vi "WVDIAL_1_AMCS_3.0.vi"() -> ()   [LabVIEW 2012]
uses:
  <vilib>/Analysis/baseanly.llb/Mean (DBL).vi
  NCAR_DIAL_Labview/AMCS_Data.vi
  AmcsUsb.dll
  <vilib>/Analysis/NI_AALBase.lvlib
panel:
  in  "scalar wait time (remove at some point)":i32=550
  in  "channel":i32=1
  in  "CH mult":dbl=1.0
  out "size(s)":i32=2241
  in  "Channels":u32=4
  in  "Data Reads":i32=52
  out "Loop Count":i32=52
  in  "TC Start":i32=2 min=1 max=1894
  in  "TC Length":i32=15 min=2 max=280
  out "TC background sub over length":cluster{dbl, dbl, dbl, dbl}(graph)={5109.382978723404, 7254.3829787234035, 34.71276595744666, -41.031914893617085}
  out "return type":i32
  out "Raw Uncorrected Return":u16[][](graph)=[[23170, 208, 128, 150, 143, 140, 160, 194, 234, 298, 421, 538, 627, 660, 684, 718, 683, 714, 813, 891, 935, 839, 807, 607, 402, 336, 228, 191, 162, 179, 228, 223, 180, 171, 156, 120, 118, 147, 143, 128, 135, 133, 141, 169, 169, 196, 157, 140, 161, 341, 3035, 18784, 23099, 23731, 21071, 6231, 426, 67, 48, 46, 51, 41, 49, 50, 54, 60, 46, 47, 40, 38, 53, 40, 37, 41, 51, 45, 57, 38, 34, 35, 35, 47, 51, 51, 57, 49, 51, 52, 33, 45, 62, 49, 34, 47, 42, 44, 35, 55, 54, 36, 40, 34, 41, 56, 52, 37, 44, 51, 52, 37, 54, 57, 45, 32, 35, 55, 44, 57, 40, 38, 37, 51, 48, 35, 55, 35, 43, 47, 48, 34, 44, 54, 44, 55, 51, 38, 46, 50, 51, 37, 44, 45, 40, 52, 42, 40, 55, 45, 40, 44, 44, 46, 38, 45, 53, 40, 52, 46, 52, 46, 42, 39, 43, 41, 34, 32, 30, 45, 46, 47, 44, 46, 37, 46, 36, 45, 49, 50, 42, 38, 45, 42, 46, 49, 51, 50, 40, 51, 36, 36, 46, 45, 37, 53, 48, 55, 51, 48, 41, 36, 47, 39, 36, 36, 36, 46, 44, 46, 43, 41, 39, 51, 51, 43, 50, 42, 44, 41, 44, 53, 54, 37, 52, 46, 46, 37, 40, 44, 42, 48, 39, 61, 40, 43, 41, 47, 42, 42, 38, 47, 34, 45, 40, 34, 44, 39, 48, 37, 53, 44, 54, 54, 48, 61, 42, 55, 39, 34, 34, 38, 38, 47, 54, 49, 44, 46, 39, 53, 49, 51, 32, 46, 39, 54, 53, 49, 34, 56, 47, 41, 47, 40, 40, 42, 34, 43, 55, 49, 47, 41, 51, 56, 63, 54, 47, 47, 44, 56, 38, 63, 42, 56, 62, 47, 37, 50, 59, 50, 42, 51, 53, 47, 43, 64, 40, 28, 41, 46, 27, 33, 56, 46, 57, 46, 58, 39, 55, 49, 49, 37, 58, 43, 38, 49, 47, 47, 33, 45, 45, 53, 42, 50, 49, 39, 43, 40, 44, 43, 49, 48, 44, 37, 42, 46, 52, 49, 45, 41, 44, 45, 36, 54, 50, 37, 34, 41, 40, 44, 37, 41, 45, 43, 56, 42, 40, 40, 34, 57, 39, 37, 42, 33, 46, 35, 40, 39, 40, 61, 38, 67, 32, 46, 61, 46, 46, 35, 42, 40, 50, 54, 47, 45, 41, 49, 47, 41, 49, 34, 46, 39, 50, 54, 45, 43, 54, 45, 50, 55, 46, 40, 37, 41, 34, 41, 46, 50, 44, 37, 55, 40, 41, 38, 37, 45, 45, 37, 37, 58, 51, 50, 39, 43, 50, 57, 49, 54, 52, 46, 43, 51, 47, 52, 45, 41, 52, 60, 51, 57, 42, 31, 46, 39, 33, 48, 42, 52, 49, 44, 51, 44, 49, 44, 39, 56, 42, 48, 41, 40, 45, 45, 40, 52, 40, 39, 38, 45, 41, 29, 44, 40, 41, 46, 50, 49, 23, 49, 52, 50, 50, 51, 50, 49, 46, 50, 39, 38, 49, 39, 50, 41, 40, 46, 36, 46, 51, 42, 37, 56, 37, 33, 43, 47, 56, 42, 48, 40, 45, 45, 49, 39, 51, 41, 43, 56, 31, 52, 35, 39, 52, 40, 44, 53, 30, 42, 48, 57, 43, 45, 39, 45, 47, 41, 52, 44, 50, 43, 52, 47, 46, 47], [23369, 189, 136, 142, 167, 134, 179, 206, 287, 391, 570, 714, 901, 981, 1009, 1038, 1068, 1177, 1297, 1480, 1537, 1540, 1386, 1167, 790, 593, 416, 343, 403, 448, 437, 400, 357, 324, 341, 292, 279, 332, 328, 343, 302, 341, 351, 440, 450, 458, 412, 358, 375, 976, 9005, 41499, 46820, 47461, 45458, 18218, 1558, 164, 60, 56, 54, 51, 52, 44, 56, 44, 48, 43, 44, 39, 37, 55, 38, 44, 44, 36, 58, 48, 44, 41, 49, 40, 50, 43, 41, 40, 46, 40, 41, 48, 55, 41, 48, 32, 47, 62, 38, 44, 40, 39, 56, 35, 37, 44, 39, 35, 33, 50, 45, 45, 43, 46, 46, 48, 41, 44, 37, 44, 49, 35, 40, 48, 55, 53, 57, 45, 43, 53, 51, 42, 46, 42, 52, 49, 46, 57, 38, 43, 52, 40, 33, 41, 46, 51, 40, 43, 42, 53, 41, 42, 42, 38, 52, 46, 43, 34, 40, 47, 43, 44, 50, 48, 45, 34, 33, 35, 46, 36, 50, 30, 51, 55, 54, 43, 41, 47, 47, 45, 57, 38, 47, 46, 58, 53, 48, 53, 45, 42, 50, 37, 52, 40, 41, 53, 57, 47, 46, 49, 46, 37, 50, 41, 38, 47, 49, 43, 58, 49, 44, 40, 41, 47, 50, 35, 47, 50, 42, 51, 29, 48, 46, 57, 34, 43, 51, 45, 47, 52, 33, 45, 46, 32, 49, 55, 45, 46, 41, 38, 53, 41, 43, 46, 40, 39, 47, 54, 44, 44, 46, 45, 42, 38, 48, 48, 42, 46, 45, 54, 46, 54, 50, 41, 50, 35, 43, 39, 40, 41, 45, 37, 40, 40, 34, 32, 48, 51, 38, 47, 46, 41, 48, 42, 50, 41, 41, 37, 32, 48, 47, 46, 46, 48, 36, 46, 55, 41, 41, 49, 40, 37, 40, 35, 45, 46, 47, 38, 54, 55, 38, 38, 45, 37, 47, 48, 46, 53, 45, 64, 39, 51, 37, 49, 53, 52, 46, 51, 42, 41, 42, 53, 47, 40, 55, 35, 43, 41, 56, 39, 51, 42, 39, 45, 38, 39, 45, 56, 51, 47, 46, 42, 40, 47, 46, 41, 30, 36, 47, 41, 46, 42, 40, 39, 58, 39, 51, 40, 35, 42, 51, 45, 36, 40, 49, 55, 39, 38, 44, 54, 60, 45, 52, 42, 48, 45, 47, 47, 38, 50, 48, 49, 43, 51, 52, 42, 36, 63, 41, 40, 47, 51, 44, 37, 47, 44, 45, 39, 44, 36, 35, 51, 56, 42, 44, 61, 35, 43, 46, 52, 53, 43, 32, 36, 40, 49, 52, 48, 35, 42, 47, 39, 44, 47, 39, 42, 42, 38, 48, 46, 48, 29, 45, 46, 41, 39, 38, 50, 46, 40, 53, 49, 51, 39, 58, 34, 41, 46, 47, 51, 52, 38, 49, 39, 51, 43, 41, 54, 49, 46, 37, 40, 38, 56, 37, 36, 48, 36, 54, 41, 40, 44, 48, 33, 39, 43, 41, 54, 42, 37, 36, 36, 30, 51, 42, 42, 53, 40, 41, 39, 49, 41, 50, 38, 53, 49, 54, 48, 59, 43, 28, 38, 39, 54, 51, 39, 48, 47, 42, 45, 40, 35, 53, 54, 53, 34, 36, 48, 37, 43, 48, 60, 51, 45, 39, 46, 45, 44, 48, 38, 52, 33, 40, 41, 37, 52, 52, 49, 54, 38, 43, 41, 53, 48, 50, 63, 57, 44, 46, 56, 35, 45], [161, 149, 145, 158, 153, 164, 145, 170, 132, 162, 165, 164, 167, 144, 148, 165, 160, 146, 144, 159, 162, 140, 181, 153, 160, 163, 158, 126, 127, 152, 160, 156, 163, 138, 172, 166, 149, 142, 144, 147, 148, 162, 134, 155, 146, 151, 159, 154, 137, 142, 148, 142, 134, 157, 144, 157, 146, 144, 140, 171, 181, 167, 151, 165, 142, 143, 160, 155, 145, 152, 139, 130, 139, 153, 168, 137, 154, 138, 146, 149, 159, 144, 150, 136, 164, 164, 151, 124, 165, 166, 149, 149, 159, 142, 147, 133, 148, 154, 155, 140, 127, 134, 147, 149, 150, 144, 146, 136, 148, 149, 175, 135, 164, 161, 162, 127, 152, 159, 131, 157, 157, 146, 154, 167, 155, 150, 148, 155, 126, 161, 174, 152, 150, 163, 152, 156, 151, 125, 152, 145, 160, 153, 138, 166, 155, 147, 152, 155, 136, 144, 156, 177, 159, 139, 148, 158, 126, 145, 148, 159, 157, 147, 159, 166, 141, 139, 156, 155, 153, 138, 144, 141, 150, 171, 148, 128, 143, 161, 149, 147, 160, 147, 141, 151, 166, 160, 155, 136, 150, 151, 157, 188, 143, 169, 144, 137, 146, 158, 157, 155, 165, 154, 173, 155, 159, 155, 147, 162, 137, 171, 161, 133, 159, 148, 142, 165, 142, 148, 146, 157, 166, 147, 153, 178, 162, 169, 146, 154, 163, 168, 139, 158, 170, 143, 162, 160, 134, 159, 151, 152, 158, 152, 136, 124, 188, 169, 142, 165, 156, 121, 147, 151, 165, 149, 139, 152, 154, 123, 127, 150, 143, 168, 167, 159, 142, 148, 153, 178, 158, 164, 171, 136, 154, 125, 128, 136, 161, 183, 163, 143, 147, 165, 129, 135, 157, 164, 142, 150, 160, 159, 163, 156, 178, 136, 158, 159, 163, 146, 175, 151, 174, 152, 133, 172, 139, 158, 166, 152, 174, 157, 158, 162, 148, 124, 160, 136, 152, 150, 156, 141, 146, 151, 153, 148, 148, 153, 153, 144, 171, 149, 165, 163, 179, 116, 142, 142, 168, 169, 139, 140, 141, 155, 151, 140, 150, 141, 151, 167, 160, 152, 153, 159, 150, 152, 169, 135, 167, 158, 152, 136, 162, 156, 166, 138, 143, 176, 166, 132, 146, 156, 150, 168, 153, 158, 132, 143, 164, 156, 140, 147, 171, 165, 130, 152, 154, 139, 153, 137, 164, 146, 145, 130, 162, 160, 152, 148, 135, 146, 174, 148, 150, 159, 156, 149, 152, 155, 158, 140, 146, 139, 159, 154, 155, 140, 152, 168, 138, 139, 157, 138, 128, 151, 159, 150, 143, 139, 163, 124, 172, 152, 165, 166, 144, 128, 156, 161, 149, 145, 137, 161, 147, 144, 135, 159, 168, 157, 141, 141, 155, 146, 148, 137, 163, 134, 138, 152, 138, 161, 141, 139, 148, 156, 139, 133, 146, 147, 144, 160, 127, 138, 174, 142, 148, 154, 140, 154, 132, 163, 164, 166, 159, 148, 120, 153, 144, 143, 156, 152, 174, 165, 149, 162, 153, 154, 168, 171, 154, 145, 177, 152, 129, 149, 159, 162, 160, 183, 143, 161, 145, 155, 175, 178, 148, 145, 156, 154, 161, 130, 142, 162, 164, 166, 163, 149, 141, 143, 172, 169, 153, 148, 144, 140, 162, 155, 150, 156, 166, 152, 148, 153, 156, 129, 146, 140, 134, 144, 151, 160, 167, 171, 136, 157, 141, 153, 178, 176, 172, 158, 167, 127], [82, 83, 88, 72, 78, 90, 58, 78, 86, 84, 68, 83, 84, 91, 85, 80, 67, 82, 62, 83, 76, 73, 90, 82, 76, 72, 79, 72, 73, 84, 73, 76, 69, 90, 74, 66, 71, 83, 84, 98, 74, 73, 86, 63, 86, 88, 80, 92, 90, 77, 74, 85, 70, 92, 68, 69, 95, 84, 96, 80, 78, 86, 75, 94, 85, 100, 93, 71, 77, 91, 91, 78, 72, 82, 73, 77, 80, 95, 98, 76, 75, 84, 77, 83, 95, 87, 80, 91, 71, 70, 105, 89, 100, 63, 90, 95, 71, 91, 68, 92, 87, 69, 79, 94, 79, 96, 91, 74, 79, 91, 73, 85, 75, 84, 72, 75, 85, 69, 90, 77, 77, 79, 80, 94, 88, 68, 70, 78, 91, 99, 82, 101, 77, 88, 93, 80, 89, 70, 78, 84, 74, 74, 80, 92, 68, 78, 66, 87, 63, 75, 82, 75, 71, 72, 97, 66, 85, 82, 87, 67, 92, 88, 84, 79, 75, 97, 71, 86, 77, 83, 89, 75, 91, 78, 76, 84, 65, 73, 77, 79, 67, 63, 87, 91, 80, 80, 98, 74, 89, 68, 95, 76, 70, 81, 60, 82, 76, 88, 85, 74, 78, 97, 86, 75, 79, 81, 76, 80, 87, 88, 75, 97, 83, 85, 93, 73, 93, 83, 72, 82, 84, 78, 83, 74, 65, 86, 82, 77, 83, 69, 96, 76, 103, 84, 79, 81, 78, 71, 72, 71, 83, 85, 90, 81, 88, 92, 79, 90, 88, 81, 72, 86, 70, 88, 79, 83, 82, 80, 73, 88, 85, 84, 92, 80, 70, 82, 75, 99, 70, 77, 82, 87, 85, 80, 84, 64, 100, 95, 88, 82, 67, 87, 83, 72, 84, 83, 90, 79, 70, 83, 84, 92, 74, 81, 60, 74, 86, 97, 82, 76, 81, 91, 93, 80, 82, 82, 69, 77, 84, 80, 103, 62, 80, 72, 79, 93, 75, 90, 90, 84, 79, 82, 69, 79, 99, 85, 85, 75, 80, 88, 69, 93, 78, 90, 79, 62, 98, 82, 94, 92, 72, 81, 84, 75, 82, 88, 67, 90, 88, 74, 75, 97, 85, 85, 79, 83, 64, 103, 92, 88, 62, 100, 94, 81, 83, 72, 74, 103, 75, 78, 94, 72, 85, 88, 84, 71, 91, 79, 78, 81, 89, 83, 76, 80, 84, 75, 77, 80, 78, 79, 75, 90, 90, 66, 76, 89, 82, 85, 100, 93, 65, 73, 89, 97, 87, 75, 96, 101, 95, 85, 92, 87, 93, 70, 78, 67, 79, 79, 77, 79, 73, 79, 64, 88, 79, 80, 70, 63, 82, 88, 83, 82, 78, 82, 100, 89, 74, 75, 76, 66, 94, 75, 81, 84, 86, 63, 82, 81, 70, 77, 83, 81, 87, 85, 70, 96, 98, 86, 86, 102, 90, 79, 77, 84, 83, 78, 92, 70, 91, 81, 92, 87, 84, 70, 80, 97, 82, 78, 68, 82, 94, 97, 80, 91, 79, 74, 66, 86, 72, 91, 87, 82, 88, 88, 83, 70, 74, 83, 96, 81, 67, 75, 86, 91, 82, 79, 90, 95, 90, 95, 89, 80, 82, 66, 86, 87, 102, 82, 77, 80, 83, 74, 80, 92, 76, 75, 67, 79, 97, 88, 76, 90, 85, 87, 76, 75, 91, 93, 74, 74, 85, 85, 88, 77, 69, 61, 79, 84, 75, 82, 73, 79, 78, 76, 77, 97, 81, 103, 84, 65]]
  in  "stop":bool
  out "Corrected Return":dbl[][](graph)=[[23125.425531914894, 163.4255319148936, 83.42553191489361, 105.42553191489361, 98.42553191489361, 95.42553191489361, 115.42553191489361, 149.4255319148936, 189.4255319148936, 253.4255319148936, 376.4255319148936, 493.4255319148936, 582.4255319148937, 615.4255319148937, 639.4255319148937, 673.4255319148937, 638.4255319148937, 669.4255319148937, 768.4255319148937, 846.4255319148937, 890.4255319148937, 794.4255319148937, 762.4255319148937, 562.4255319148937, 357.4255319148936, 291.4255319148936, 183.4255319148936, 146.4255319148936, 117.42553191489361, 134.4255319148936, 183.4255319148936, 178.4255319148936, 135.4255319148936, 126.42553191489361, 111.42553191489361, 75.42553191489361, 73.42553191489361, 102.42553191489361, 98.42553191489361, 83.42553191489361, 90.42553191489361, 88.42553191489361, 96.42553191489361, 124.42553191489361, 124.42553191489361, 151.4255319148936, 112.42553191489361, 95.42553191489361, 116.42553191489361, 296.4255319148936, 2990.425531914894, 18739.425531914894, 23054.425531914894, 23686.425531914894, 21026.425531914894, 6186.425531914893, 381.4255319148936, 22.425531914893618, 3.425531914893618, 1.425531914893618, 6.425531914893618, -3.574468085106382, 4.425531914893618, 5.425531914893618, 9.425531914893618, 15.425531914893618, 1.425531914893618, 2.425531914893618, -4.574468085106382, -6.574468085106382, 8.425531914893618, -4.574468085106382, -7.574468085106382, -3.574468085106382, 6.425531914893618, 0.4255319148936181, 12.425531914893618, -6.574468085106382, -10.574468085106382, -9.574468085106382, -9.574468085106382, 2.425531914893618, 6.425531914893618, 6.425531914893618, 12.425531914893618, 4.425531914893618, 6.425531914893618, 7.425531914893618, -11.574468085106382, 0.4255319148936181, 17.425531914893618, 4.425531914893618, -10.574468085106382, 2.425531914893618, -2.574468085106382, -0.5744680851063819, -9.574468085106382, 10.425531914893618, 9.425531914893618, -8.574468085106382, -4.574468085106382, -10.574468085106382, -3.574468085106382, 11.425531914893618, 7.425531914893618, -7.574468085106382, -0.5744680851063819, 6.425531914893618, 7.425531914893618, -7.574468085106382, 9.425531914893618, 12.425531914893618, 0.4255319148936181, -12.574468085106382, -9.574468085106382, 10.425531914893618, -0.5744680851063819, 12.425531914893618, -4.574468085106382, -6.574468085106382, -7.574468085106382, 6.425531914893618, 3.425531914893618, -9.574468085106382, 10.425531914893618, -9.574468085106382, -1.574468085106382, 2.425531914893618, 3.425531914893618, -10.574468085106382, -0.5744680851063819, 9.425531914893618, -0.5744680851063819, 10.425531914893618, 6.425531914893618, -6.574468085106382, 1.425531914893618, 5.425531914893618, 6.425531914893618, -7.574468085106382, -0.5744680851063819, 0.4255319148936181, -4.574468085106382, 7.425531914893618, -2.574468085106382, -4.574468085106382, 10.425531914893618, 0.4255319148936181, -4.574468085106382, -0.5744680851063819, -0.5744680851063819, 1.425531914893618, -6.574468085106382, 0.4255319148936181, 8.425531914893618, -4.574468085106382, 7.425531914893618, 1.425531914893618, 7.425531914893618, 1.425531914893618, -2.574468085106382, -5.574468085106382, -1.574468085106382, -3.574468085106382, -10.574468085106382, -12.574468085106382, -14.574468085106382, 0.4255319148936181, 1.425531914893618, 2.425531914893618, -0.5744680851063819, 1.425531914893618, -7.574468085106382, 1.425531914893618, -8.574468085106382, 0.4255319148936181, 4.425531914893618, 5.425531914893618, -2.574468085106382, -6.574468085106382, 0.4255319148936181, -2.574468085106382, 1.425531914893618, 4.425531914893618, 6.425531914893618, 5.425531914893618, -4.574468085106382, 6.425531914893618, -8.574468085106382, -8.574468085106382, 1.425531914893618, 0.4255319148936181, -7.574468085106382, 8.425531914893618, 3.425531914893618, 10.425531914893618, 6.425531914893618, 3.425531914893618, -3.574468085106382, -8.574468085106382, 2.425531914893618, -5.574468085106382, -8.574468085106382, -8.574468085106382, -8.574468085106382, 1.425531914893618, -0.5744680851063819, 1.425531914893618, -1.574468085106382, -3.574468085106382, -5.574468085106382, 6.425531914893618, 6.425531914893618, -1.574468085106382, 5.425531914893618, -2.574468085106382, -0.5744680851063819, -3.574468085106382, -0.5744680851063819, 8.425531914893618, 9.425531914893618, -7.574468085106382, 7.425531914893618, 1.425531914893618, 1.425531914893618, -7.574468085106382, -4.574468085106382, -0.5744680851063819, -2.574468085106382, 3.425531914893618, -5.574468085106382, 16.425531914893618, -4.574468085106382, -1.574468085106382, -3.574468085106382, 2.425531914893618, -2.574468085106382, -2.574468085106382, -6.574468085106382, 2.425531914893618, -10.574468085106382, 0.4255319148936181, -4.574468085106382, -10.574468085106382, -0.5744680851063819, -5.574468085106382, 3.425531914893618, -7.574468085106382, 8.425531914893618, -0.5744680851063819, 9.425531914893618, 9.425531914893618, 3.425531914893618, 16.425531914893618, -2.574468085106382, 10.425531914893618, -5.574468085106382, -10.574468085106382, -10.574468085106382, -6.574468085106382, -6.574468085106382, 2.425531914893618, 9.425531914893618, 4.425531914893618, -0.5744680851063819, 1.425531914893618, -5.574468085106382, 8.425531914893618, 4.425531914893618, 6.425531914893618, -12.574468085106382, 1.425531914893618, -5.574468085106382, 9.425531914893618, 8.425531914893618, 4.425531914893618, -10.574468085106382, 11.425531914893618, 2.425531914893618, -3.574468085106382, 2.425531914893618, -4.574468085106382, -4.574468085106382, -2.574468085106382, -10.574468085106382, -1.574468085106382, 10.425531914893618, 4.425531914893618, 2.425531914893618, -3.574468085106382, 6.425531914893618, 11.425531914893618, 18.425531914893618, 9.425531914893618, 2.425531914893618, 2.425531914893618, -0.5744680851063819, 11.425531914893618, -6.574468085106382, 18.425531914893618, -2.574468085106382, 11.425531914893618, 17.425531914893618, 2.425531914893618, -7.574468085106382, 5.425531914893618, 14.425531914893618, 5.425531914893618, -2.574468085106382, 6.425531914893618, 8.425531914893618, 2.425531914893618, -1.574468085106382, 19.425531914893618, -4.574468085106382, -16.574468085106382, -3.574468085106382, 1.425531914893618, -17.574468085106382, -11.574468085106382, 11.425531914893618, 1.425531914893618, 12.425531914893618, 1.425531914893618, 13.425531914893618, -5.574468085106382, 10.425531914893618, 4.425531914893618, 4.425531914893618, -7.574468085106382, 13.425531914893618, -1.574468085106382, -6.574468085106382, 4.425531914893618, 2.425531914893618, 2.425531914893618, -11.574468085106382, 0.4255319148936181, 0.4255319148936181, 8.425531914893618, -2.574468085106382, 5.425531914893618, 4.425531914893618, -5.574468085106382, -1.574468085106382, -4.574468085106382, -0.5744680851063819, -1.574468085106382, 4.425531914893618, 3.425531914893618, -0.5744680851063819, -7.574468085106382, -2.574468085106382, 1.425531914893618, 7.425531914893618, 4.425531914893618, 0.4255319148936181, -3.574468085106382, -0.5744680851063819, 0.4255319148936181, -8.574468085106382, 9.425531914893618, 5.425531914893618, -7.574468085106382, -10.574468085106382, -3.574468085106382, -4.574468085106382, -0.5744680851063819, -7.574468085106382, -3.574468085106382, 0.4255319148936181, -1.574468085106382, 11.425531914893618, -2.574468085106382, -4.574468085106382, -4.574468085106382, -10.574468085106382, 12.425531914893618, -5.574468085106382, -7.574468085106382, -2.574468085106382, -11.574468085106382, 1.425531914893618, -9.574468085106382, -4.574468085106382, -5.574468085106382, -4.574468085106382, 16.425531914893618, -6.574468085106382, 22.425531914893618, -12.574468085106382, 1.425531914893618, 16.425531914893618, 1.425531914893618, 1.425531914893618, -9.574468085106382, -2.574468085106382, -4.574468085106382, 5.425531914893618, 9.425531914893618, 2.425531914893618, 0.4255319148936181, -3.574468085106382, 4.425531914893618, 2.425531914893618, -3.574468085106382, 4.425531914893618, -10.574468085106382, 1.425531914893618, -5.574468085106382, 5.425531914893618, 9.425531914893618, 0.4255319148936181, -1.574468085106382, 9.425531914893618, 0.4255319148936181, 5.425531914893618, 10.425531914893618, 1.425531914893618, -4.574468085106382, -7.574468085106382, -3.574468085106382, -10.574468085106382, -3.574468085106382, 1.425531914893618, 5.425531914893618, -0.5744680851063819, -7.574468085106382, 10.425531914893618, -4.574468085106382, -3.574468085106382, -6.574468085106382, -7.574468085106382, 0.4255319148936181, 0.4255319148936181, -7.574468085106382, -7.574468085106382, 13.425531914893618, 6.425531914893618, 5.425531914893618, -5.574468085106382, -1.574468085106382, 5.425531914893618, 12.425531914893618, 4.425531914893618, 9.425531914893618, 7.425531914893618, 1.425531914893618, -1.574468085106382, 6.425531914893618, 2.425531914893618, 7.425531914893618, 0.4255319148936181, -3.574468085106382, 7.425531914893618, 15.425531914893618, 6.425531914893618, 12.425531914893618, -2.574468085106382, -13.574468085106382, 1.425531914893618, -5.574468085106382, -11.574468085106382, 3.425531914893618, -2.574468085106382, 7.425531914893618, 4.425531914893618, -0.5744680851063819, 6.425531914893618, -0.5744680851063819, 4.425531914893618, -0.5744680851063819, -5.574468085106382, 11.425531914893618, -2.574468085106382, 3.425531914893618, -3.574468085106382, -4.574468085106382, 0.4255319148936181, 0.4255319148936181, -4.574468085106382, 7.425531914893618, -4.574468085106382, -5.574468085106382, -6.574468085106382, 0.4255319148936181, -3.574468085106382, -15.574468085106382, -0.5744680851063819, -4.574468085106382, -3.574468085106382, 1.425531914893618, 5.425531914893618, 4.425531914893618, -21.574468085106382, 4.425531914893618, 7.425531914893618, 5.425531914893618, 5.425531914893618, 6.425531914893618, 5.425531914893618, 4.425531914893618, 1.425531914893618, 5.425531914893618, -5.574468085106382, -6.574468085106382, 4.425531914893618, -5.574468085106382, 5.425531914893618, -3.574468085106382, -4.574468085106382, 1.425531914893618, -8.574468085106382, 1.425531914893618, 6.425531914893618, -2.574468085106382, -7.574468085106382, 11.425531914893618, -7.574468085106382, -11.574468085106382, -1.574468085106382, 2.425531914893618, 11.425531914893618, -2.574468085106382, 3.425531914893618, -4.574468085106382, 0.4255319148936181, 0.4255319148936181, 4.425531914893618, -5.574468085106382, 6.425531914893618, -3.574468085106382, -1.574468085106382, 11.425531914893618, -13.574468085106382, 7.425531914893618, -9.574468085106382, -5.574468085106382, 7.425531914893618, -4.574468085106382, -0.5744680851063819, 8.425531914893618, -14.574468085106382, -2.574468085106382, 3.425531914893618, 12.425531914893618, -1.574468085106382, 0.4255319148936181, -5.574468085106382, 0.4255319148936181, 2.425531914893618, -3.574468085106382, 7.425531914893618, -0.5744680851063819, 5.425531914893618, -1.574468085106382, 7.425531914893618, 2.425531914893618, 1.425531914893618, 2.425531914893618], [23324.425531914894, 144.4255319148936, 91.42553191489361, 97.42553191489361, 122.42553191489361, 89.42553191489361, 134.4255319148936, 161.4255319148936, 242.4255319148936, 346.4255319148936, 525.4255319148937, 669.4255319148937, 856.4255319148937, 936.4255319148937, 964.4255319148937, 993.4255319148937, 1023.4255319148937, 1132.4255319148936, 1252.4255319148936, 1435.4255319148936, 1492.4255319148936, 1495.4255319148936, 1341.4255319148936, 1122.4255319148936, 745.4255319148937, 548.4255319148937, 371.4255319148936, 298.4255319148936, 358.4255319148936, 403.4255319148936, 392.4255319148936, 355.4255319148936, 312.4255319148936, 279.4255319148936, 296.4255319148936, 247.4255319148936, 234.4255319148936, 287.4255319148936, 283.4255319148936, 298.4255319148936, 257.4255319148936, 296.4255319148936, 306.4255319148936, 395.4255319148936, 405.4255319148936, 413.4255319148936, 367.4255319148936, 313.4255319148936, 330.4255319148936, 931.4255319148937, 8960.425531914894, 41454.425531914894, 46775.425531914894, 47416.425531914894, 45413.425531914894, 18173.425531914894, 1513.4255319148936, 119.42553191489361, 15.425531914893618, 11.425531914893618, 9.425531914893618, 6.425531914893618, 7.425531914893618, -0.5744680851063819, 11.425531914893618, -0.5744680851063819, 3.425531914893618, -1.574468085106382, -0.5744680851063819, -5.574468085106382, -7.574468085106382, 10.425531914893618, -6.574468085106382, -0.5744680851063819, -0.5744680851063819, -8.574468085106382, 13.425531914893618, 3.425531914893618, -0.5744680851063819, -3.574468085106382, 4.425531914893618, -4.574468085106382, 5.425531914893618, -1.574468085106382, -3.574468085106382, -4.574468085106382, 1.425531914893618, -4.574468085106382, -3.574468085106382, 3.425531914893618, 10.425531914893618, -3.574468085106382, 3.425531914893618, -12.574468085106382, 2.425531914893618, 17.425531914893618, -6.574468085106382, -0.5744680851063819, -4.574468085106382, -5.574468085106382, 11.425531914893618, -9.574468085106382, -7.574468085106382, -0.5744680851063819, -5.574468085106382, -9.574468085106382, -11.574468085106382, 5.425531914893618, 0.4255319148936181, 0.4255319148936181, -1.574468085106382, 1.425531914893618, 1.425531914893618, 3.425531914893618, -3.574468085106382, -0.5744680851063819, -7.574468085106382, -0.5744680851063819, 4.425531914893618, -9.574468085106382, -4.574468085106382, 3.425531914893618, 10.425531914893618, 8.425531914893618, 12.425531914893618, 0.4255319148936181, -1.574468085106382, 8.425531914893618, 6.425531914893618, -2.574468085106382, 1.425531914893618, -2.574468085106382, 7.425531914893618, 4.425531914893618, 1.425531914893618, 12.425531914893618, -6.574468085106382, -1.574468085106382, 7.425531914893618, -4.574468085106382, -11.574468085106382, -3.574468085106382, 1.425531914893618, 6.425531914893618, -4.574468085106382, -1.574468085106382, -2.574468085106382, 8.425531914893618, -3.574468085106382, -2.574468085106382, -2.574468085106382, -6.574468085106382, 7.425531914893618, 1.425531914893618, -1.574468085106382, -10.574468085106382, -4.574468085106382, 2.425531914893618, -1.574468085106382, -0.5744680851063819, 5.425531914893618, 3.425531914893618, 0.4255319148936181, -10.574468085106382, -11.574468085106382, -9.574468085106382, 1.425531914893618, -8.574468085106382, 5.425531914893618, -14.574468085106382, 6.425531914893618, 10.425531914893618, 9.425531914893618, -1.574468085106382, -3.574468085106382, 2.425531914893618, 2.425531914893618, 0.4255319148936181, 12.425531914893618, -6.574468085106382, 2.425531914893618, 1.425531914893618, 13.425531914893618, 8.425531914893618, 3.425531914893618, 8.425531914893618, 0.4255319148936181, -2.574468085106382, 5.425531914893618, -7.574468085106382, 7.425531914893618, -4.574468085106382, -3.574468085106382, 8.425531914893618, 12.425531914893618, 2.425531914893618, 1.425531914893618, 4.425531914893618, 1.425531914893618, -7.574468085106382, 5.425531914893618, -3.574468085106382, -6.574468085106382, 2.425531914893618, 4.425531914893618, -1.574468085106382, 13.425531914893618, 4.425531914893618, -0.5744680851063819, -4.574468085106382, -3.574468085106382, 2.425531914893618, 5.425531914893618, -9.574468085106382, 2.425531914893618, 5.425531914893618, -2.574468085106382, 6.425531914893618, -15.574468085106382, 3.425531914893618, 1.425531914893618, 12.425531914893618, -10.574468085106382, -1.574468085106382, 6.425531914893618, 0.4255319148936181, 2.425531914893618, 7.425531914893618, -11.574468085106382, 0.4255319148936181, 1.425531914893618, -12.574468085106382, 4.425531914893618, 10.425531914893618, 0.4255319148936181, 1.425531914893618, -3.574468085106382, -6.574468085106382, 8.425531914893618, -3.574468085106382, -1.574468085106382, 1.425531914893618, -4.574468085106382, -5.574468085106382, 2.425531914893618, 9.425531914893618, -0.5744680851063819, -0.5744680851063819, 1.425531914893618, 0.4255319148936181, -2.574468085106382, -6.574468085106382, 3.425531914893618, 3.425531914893618, -2.574468085106382, 1.425531914893618, 0.4255319148936181, 9.425531914893618, 1.425531914893618, 9.425531914893618, 5.425531914893618, -3.574468085106382, 5.425531914893618, -9.574468085106382, -1.574468085106382, -5.574468085106382, -4.574468085106382, -3.574468085106382, 0.4255319148936181, -7.574468085106382, -4.574468085106382, -4.574468085106382, -10.574468085106382, -12.574468085106382, 3.425531914893618, 6.425531914893618, -6.574468085106382, 2.425531914893618, 1.425531914893618, -3.574468085106382, 3.425531914893618, -2.574468085106382, 5.425531914893618, -3.574468085106382, -3.574468085106382, -7.574468085106382, -12.574468085106382, 3.425531914893618, 2.425531914893618, 1.425531914893618, 1.425531914893618, 3.425531914893618, -8.574468085106382, 1.425531914893618, 10.425531914893618, -3.574468085106382, -3.574468085106382, 4.425531914893618, -4.574468085106382, -7.574468085106382, -4.574468085106382, -9.574468085106382, 0.4255319148936181, 1.425531914893618, 2.425531914893618, -6.574468085106382, 9.425531914893618, 10.425531914893618, -6.574468085106382, -6.574468085106382, 0.4255319148936181, -7.574468085106382, 2.425531914893618, 3.425531914893618, 1.425531914893618, 8.425531914893618, 0.4255319148936181, 19.425531914893618, -5.574468085106382, 6.425531914893618, -7.574468085106382, 4.425531914893618, 8.425531914893618, 7.425531914893618, 1.425531914893618, 6.425531914893618, -2.574468085106382, -3.574468085106382, -2.574468085106382, 8.425531914893618, 2.425531914893618, -4.574468085106382, 10.425531914893618, -9.574468085106382, -1.574468085106382, -3.574468085106382, 11.425531914893618, -5.574468085106382, 6.425531914893618, -2.574468085106382, -5.574468085106382, 0.4255319148936181, -6.574468085106382, -5.574468085106382, 0.4255319148936181, 11.425531914893618, 6.425531914893618, 2.425531914893618, 1.425531914893618, -2.574468085106382, -4.574468085106382, 2.425531914893618, 1.425531914893618, -3.574468085106382, -14.574468085106382, -8.574468085106382, 2.425531914893618, -3.574468085106382, 1.425531914893618, -2.574468085106382, -4.574468085106382, -5.574468085106382, 13.425531914893618, -5.574468085106382, 6.425531914893618, -4.574468085106382, -9.574468085106382, -2.574468085106382, 6.425531914893618, 0.4255319148936181, -8.574468085106382, -4.574468085106382, 4.425531914893618, 10.425531914893618, -5.574468085106382, -6.574468085106382, -0.5744680851063819, 9.425531914893618, 15.425531914893618, 0.4255319148936181, 7.425531914893618, -2.574468085106382, 3.425531914893618, 0.4255319148936181, 2.425531914893618, 2.425531914893618, -6.574468085106382, 5.425531914893618, 3.425531914893618, 4.425531914893618, -1.574468085106382, 6.425531914893618, 7.425531914893618, -2.574468085106382, -8.574468085106382, 18.425531914893618, -3.574468085106382, -4.574468085106382, 2.425531914893618, 6.425531914893618, -0.5744680851063819, -7.574468085106382, 2.425531914893618, -0.5744680851063819, 0.4255319148936181, -5.574468085106382, -0.5744680851063819, -8.574468085106382, -9.574468085106382, 6.425531914893618, 11.425531914893618, -2.574468085106382, -0.5744680851063819, 16.425531914893618, -9.574468085106382, -1.574468085106382, 1.425531914893618, 7.425531914893618, 8.425531914893618, -1.574468085106382, -12.574468085106382, -8.574468085106382, -4.574468085106382, 4.425531914893618, 7.425531914893618, 3.425531914893618, -9.574468085106382, -2.574468085106382, 2.425531914893618, -5.574468085106382, -0.5744680851063819, 2.425531914893618, -5.574468085106382, -2.574468085106382, -2.574468085106382, -6.574468085106382, 3.425531914893618, 1.425531914893618, 3.425531914893618, -15.574468085106382, 0.4255319148936181, 1.425531914893618, -3.574468085106382, -5.574468085106382, -6.574468085106382, 5.425531914893618, 1.425531914893618, -4.574468085106382, 8.425531914893618, 4.425531914893618, 6.425531914893618, -5.574468085106382, 13.425531914893618, -10.574468085106382, -3.574468085106382, 1.425531914893618, 2.425531914893618, 6.425531914893618, 7.425531914893618, -6.574468085106382, 4.425531914893618, -5.574468085106382, 6.425531914893618, -1.574468085106382, -3.574468085106382, 9.425531914893618, 4.425531914893618, 1.425531914893618, -7.574468085106382, -4.574468085106382, -6.574468085106382, 11.425531914893618, -7.574468085106382, -8.574468085106382, 3.425531914893618, -8.574468085106382, 9.425531914893618, -3.574468085106382, -4.574468085106382, -0.5744680851063819, 3.425531914893618, -11.574468085106382, -5.574468085106382, -1.574468085106382, -3.574468085106382, 9.425531914893618, -2.574468085106382, -7.574468085106382, -8.574468085106382, -8.574468085106382, -14.574468085106382, 6.425531914893618, -2.574468085106382, -2.574468085106382, 8.425531914893618, -4.574468085106382, -3.574468085106382, -5.574468085106382, 4.425531914893618, -3.574468085106382, 5.425531914893618, -6.574468085106382, 8.425531914893618, 4.425531914893618, 9.425531914893618, 3.425531914893618, 14.425531914893618, -1.574468085106382, -16.574468085106382, -6.574468085106382, -5.574468085106382, 9.425531914893618, 6.425531914893618, -5.574468085106382, 3.425531914893618, 2.425531914893618, -2.574468085106382, 0.4255319148936181, -4.574468085106382, -9.574468085106382, 8.425531914893618, 9.425531914893618, 8.425531914893618, -10.574468085106382, -8.574468085106382, 3.425531914893618, -7.574468085106382, -1.574468085106382, 3.425531914893618, 15.425531914893618, 6.425531914893618, 0.4255319148936181, -5.574468085106382, 1.425531914893618, 0.4255319148936181, -0.5744680851063819, 3.425531914893618, -6.574468085106382, 7.425531914893618, -11.574468085106382, -4.574468085106382, -3.574468085106382, -7.574468085106382, 7.425531914893618, 7.425531914893618, 4.425531914893618, 9.425531914893618, -6.574468085106382, -1.574468085106382, -3.574468085106382, 8.425531914893618, 3.425531914893618, 5.425531914893618, 18.425531914893618, 12.425531914893618, -0.5744680851063819, 1.425531914893618, 11.425531914893618, -9.574468085106382, 0.4255319148936181], [7.180851063829778, -4.819148936170222, -8.819148936170222, 4.180851063829778, -0.8191489361702224, 10.180851063829778, -8.819148936170222, 16.180851063829778, -21.819148936170222, 8.180851063829778, 11.180851063829778, 10.180851063829778, 13.180851063829778, -9.819148936170222, -5.819148936170222, 11.180851063829778, 6.180851063829778, -7.819148936170222, -9.819148936170222, 5.180851063829778, 8.180851063829778, -13.819148936170222, 27.180851063829778, -0.8191489361702224, 6.180851063829778, 9.180851063829778, 4.180851063829778, -27.819148936170222, -26.819148936170222, -1.8191489361702224, 6.180851063829778, 2.1808510638297776, 9.180851063829778, -15.819148936170222, 18.180851063829778, 12.180851063829778, -4.819148936170222, -11.819148936170222, -9.819148936170222, -6.819148936170222, -5.819148936170222, 8.180851063829778, -19.819148936170222, 1.1808510638297776, -7.819148936170222, -2.8191489361702224, 5.180851063829778, 0.18085106382977756, -16.819148936170222, -11.819148936170222, -5.819148936170222, -11.819148936170222, -19.819148936170222, 3.1808510638297776, -9.819148936170222, 3.1808510638297776, -7.819148936170222, -9.819148936170222, -13.819148936170222, 17.180851063829778, 27.180851063829778, 13.180851063829778, -2.8191489361702224, 11.180851063829778, -11.819148936170222, -10.819148936170222, 6.180851063829778, 1.1808510638297776, -8.819148936170222, -1.8191489361702224, -14.819148936170222, -23.819148936170222, -14.819148936170222, -0.8191489361702224, 14.180851063829778, -16.819148936170222, 0.18085106382977756, -15.819148936170222, -7.819148936170222, -4.819148936170222, 5.180851063829778, -9.819148936170222, -3.8191489361702224, -17.819148936170222, 10.180851063829778, 10.180851063829778, -2.8191489361702224, -29.819148936170222, 11.180851063829778, 12.180851063829778, -4.819148936170222, -4.819148936170222, 5.180851063829778, -11.819148936170222, -6.819148936170222, -20.819148936170222, -5.819148936170222, 0.18085106382977756, 1.1808510638297776, -13.819148936170222, -26.819148936170222, -19.819148936170222, -6.819148936170222, -4.819148936170222, -3.8191489361702224, -9.819148936170222, -7.819148936170222, -17.819148936170222, -5.819148936170222, -4.819148936170222, 21.180851063829778, -18.819148936170222, 10.180851063829778, 7.180851063829778, 8.180851063829778, -26.819148936170222, -1.8191489361702224, 5.180851063829778, -22.819148936170222, 3.1808510638297776, 3.1808510638297776, -7.819148936170222, 0.18085106382977756, 13.180851063829778, 1.1808510638297776, -3.8191489361702224, -5.819148936170222, 1.1808510638297776, -27.819148936170222, 7.180851063829778, 20.180851063829778, -1.8191489361702224, -3.8191489361702224, 9.180851063829778, -1.8191489361702224, 2.1808510638297776, -2.8191489361702224, -28.819148936170222, -1.8191489361702224, -8.819148936170222, 6.180851063829778, -0.8191489361702224, -15.819148936170222, 12.180851063829778, 1.1808510638297776, -6.819148936170222, -1.8191489361702224, 1.1808510638297776, -17.819148936170222, -9.819148936170222, 2.1808510638297776, 23.180851063829778, 5.180851063829778, -14.819148936170222, -5.819148936170222, 4.180851063829778, -27.819148936170222, -8.819148936170222, -5.819148936170222, 5.180851063829778, 3.1808510638297776, -6.819148936170222, 5.180851063829778, 12.180851063829778, -12.819148936170222, -14.819148936170222, 2.1808510638297776, 1.1808510638297776, -0.8191489361702224, -15.819148936170222, -9.819148936170222, -12.819148936170222, -3.8191489361702224, 17.180851063829778, -5.819148936170222, -25.819148936170222, -10.819148936170222, 7.180851063829778, -4.819148936170222, -6.819148936170222, 6.180851063829778, -6.819148936170222, -12.819148936170222, -2.8191489361702224, 12.180851063829778, 6.180851063829778, 1.1808510638297776, -17.819148936170222, -3.8191489361702224, -2.8191489361702224, 3.1808510638297776, 34.18085106382978, -10.819148936170222, 15.180851063829778, -9.819148936170222, -16.819148936170222, -7.819148936170222, 4.180851063829778, 3.1808510638297776, 1.1808510638297776, 11.180851063829778, 0.18085106382977756, 19.180851063829778, 1.1808510638297776, 5.180851063829778, 1.1808510638297776, -6.819148936170222, 8.180851063829778, -16.819148936170222, 17.180851063829778, 7.180851063829778, -20.819148936170222, 5.180851063829778, -5.819148936170222, -11.819148936170222, 11.180851063829778, -11.819148936170222, -5.819148936170222, -7.819148936170222, 3.1808510638297776, 12.180851063829778, -6.819148936170222, -0.8191489361702224, 24.180851063829778, 8.180851063829778, 15.180851063829778, -7.819148936170222, 0.18085106382977756, 9.180851063829778, 14.180851063829778, -14.819148936170222, 4.180851063829778, 16.180851063829778, -10.819148936170222, 8.180851063829778, 6.180851063829778, -19.819148936170222, 5.180851063829778, -2.8191489361702224, -1.8191489361702224, 4.180851063829778, -1.8191489361702224, -17.819148936170222, -29.819148936170222, 34.18085106382978, 15.180851063829778, -11.819148936170222, 11.180851063829778, 2.1808510638297776, -32.81914893617022, -6.819148936170222, -2.8191489361702224, 11.180851063829778, -4.819148936170222, -14.819148936170222, -1.8191489361702224, 0.18085106382977756, -30.819148936170222, -26.819148936170222, -3.8191489361702224, -10.819148936170222, 14.180851063829778, 13.180851063829778, 5.180851063829778, -11.819148936170222, -5.819148936170222, -0.8191489361702224, 24.180851063829778, 4.180851063829778, 10.180851063829778, 17.180851063829778, -17.819148936170222, 0.18085106382977756, -28.819148936170222, -25.819148936170222, -17.819148936170222, 7.180851063829778, 29.180851063829778, 9.180851063829778, -10.819148936170222, -6.819148936170222, 11.180851063829778, -24.819148936170222, -18.819148936170222, 3.1808510638297776, 10.180851063829778, -11.819148936170222, -3.8191489361702224, 6.180851063829778, 5.180851063829778, 9.180851063829778, 2.1808510638297776, 24.180851063829778, -17.819148936170222, 4.180851063829778, 5.180851063829778, 9.180851063829778, -7.819148936170222, 21.180851063829778, -2.8191489361702224, 20.180851063829778, -1.8191489361702224, -20.819148936170222, 18.180851063829778, -14.819148936170222, 4.180851063829778, 12.180851063829778, -1.8191489361702224, 20.180851063829778, 3.1808510638297776, 4.180851063829778, 8.180851063829778, -5.819148936170222, -29.819148936170222, 6.180851063829778, -17.819148936170222, -1.8191489361702224, -3.8191489361702224, 2.1808510638297776, -12.819148936170222, -7.819148936170222, -2.8191489361702224, -0.8191489361702224, -5.819148936170222, -5.819148936170222, -0.8191489361702224, -0.8191489361702224, -9.819148936170222, 17.180851063829778, -4.819148936170222, 11.180851063829778, 9.180851063829778, 25.180851063829778, -37.81914893617022, -11.819148936170222, -11.819148936170222, 14.180851063829778, 15.180851063829778, -14.819148936170222, -13.819148936170222, -12.819148936170222, 1.1808510638297776, -2.8191489361702224, -13.819148936170222, -3.8191489361702224, -12.819148936170222, -2.8191489361702224, 13.180851063829778, 6.180851063829778, -1.8191489361702224, -0.8191489361702224, 5.180851063829778, -3.8191489361702224, -1.8191489361702224, 15.180851063829778, -18.819148936170222, 13.180851063829778, 4.180851063829778, -1.8191489361702224, -17.819148936170222, 8.180851063829778, 2.1808510638297776, 12.180851063829778, -15.819148936170222, -10.819148936170222, 22.180851063829778, 12.180851063829778, -21.819148936170222, -7.819148936170222, 2.1808510638297776, -3.8191489361702224, 14.180851063829778, -0.8191489361702224, 4.180851063829778, -21.819148936170222, -10.819148936170222, 10.180851063829778, 2.1808510638297776, -13.819148936170222, -6.819148936170222, 17.180851063829778, 11.180851063829778, -23.819148936170222, -1.8191489361702224, 0.18085106382977756, -14.819148936170222, -0.8191489361702224, -16.819148936170222, 10.180851063829778, -7.819148936170222, -8.819148936170222, -23.819148936170222, 8.180851063829778, 6.180851063829778, -1.8191489361702224, -5.819148936170222, -18.819148936170222, -7.819148936170222, 20.180851063829778, -5.819148936170222, -3.8191489361702224, 5.180851063829778, 2.1808510638297776, -4.819148936170222, -1.8191489361702224, 1.1808510638297776, 4.180851063829778, -13.819148936170222, -7.819148936170222, -14.819148936170222, 5.180851063829778, 0.18085106382977756, 1.1808510638297776, -13.819148936170222, -1.8191489361702224, 14.180851063829778, -15.819148936170222, -14.819148936170222, 3.1808510638297776, -15.819148936170222, -25.819148936170222, -2.8191489361702224, 5.180851063829778, -3.8191489361702224, -10.819148936170222, -14.819148936170222, 9.180851063829778, -29.819148936170222, 18.180851063829778, -1.8191489361702224, 11.180851063829778, 12.180851063829778, -9.819148936170222, -25.819148936170222, 2.1808510638297776, 7.180851063829778, -4.819148936170222, -8.819148936170222, -16.819148936170222, 7.180851063829778, -6.819148936170222, -9.819148936170222, -18.819148936170222, 5.180851063829778, 14.180851063829778, 3.1808510638297776, -12.819148936170222, -12.819148936170222, 1.1808510638297776, -7.819148936170222, -5.819148936170222, -16.819148936170222, 9.180851063829778, -19.819148936170222, -15.819148936170222, -1.8191489361702224, -15.819148936170222, 7.180851063829778, -12.819148936170222, -14.819148936170222, -5.819148936170222, 2.1808510638297776, -14.819148936170222, -20.819148936170222, -7.819148936170222, -6.819148936170222, -9.819148936170222, 6.180851063829778, -26.819148936170222, -15.819148936170222, 20.180851063829778, -11.819148936170222, -5.819148936170222, 0.18085106382977756, -13.819148936170222, 0.18085106382977756, -21.819148936170222, 9.180851063829778, 10.180851063829778, 12.180851063829778, 5.180851063829778, -5.819148936170222, -33.81914893617022, -0.8191489361702224, -9.819148936170222, -10.819148936170222, 2.1808510638297776, -1.8191489361702224, 20.180851063829778, 11.180851063829778, -4.819148936170222, 8.180851063829778, -0.8191489361702224, 0.18085106382977756, 14.180851063829778, 17.180851063829778, 0.18085106382977756, -8.819148936170222, 23.180851063829778, -1.8191489361702224, -24.819148936170222, -4.819148936170222, 5.180851063829778, 8.180851063829778, 6.180851063829778, 29.180851063829778, -10.819148936170222, 7.180851063829778, -8.819148936170222, 1.1808510638297776, 21.180851063829778, 24.180851063829778, -5.819148936170222, -8.819148936170222, 2.1808510638297776, 0.18085106382977756, 7.180851063829778, -23.819148936170222, -11.819148936170222, 8.180851063829778, 10.180851063829778, 12.180851063829778, 9.180851063829778, -4.819148936170222, -12.819148936170222, -10.819148936170222, 18.180851063829778, 15.180851063829778, -0.8191489361702224, -5.819148936170222, -9.819148936170222, -13.819148936170222, 8.180851063829778, 1.1808510638297776, -3.8191489361702224, 2.1808510638297776, 12.180851063829778, -1.8191489361702224, -5.819148936170222, -0.8191489361702224, 2.1808510638297776, -24.819148936170222, -7.819148936170222, -13.819148936170222, -19.819148936170222, -9.819148936170222, -2.8191489361702224, 6.180851063829778, 13.180851063829778, 17.180851063829778, -17.819148936170222, 3.1808510638297776, -12.819148936170222, -0.8191489361702224, 24.180851063829778, 22.180851063829778, 18.180851063829778, 4.180851063829778, 13.180851063829778, -26.819148936170222], [-0.20212765957447232, 0.7978723404255277, 5.797872340425528, -10.202127659574472, -4.202127659574472, 7.797872340425528, -24.202127659574472, -4.202127659574472, 3.7978723404255277, 1.7978723404255277, -14.202127659574472, 0.7978723404255277, 1.7978723404255277, 8.797872340425528, 2.7978723404255277, -2.2021276595744723, -15.202127659574472, -0.20212765957447232, -20.202127659574472, 0.7978723404255277, -6.202127659574472, -9.202127659574472, 7.797872340425528, -0.20212765957447232, -6.202127659574472, -10.202127659574472, -3.2021276595744723, -10.202127659574472, -9.202127659574472, 1.7978723404255277, -9.202127659574472, -6.202127659574472, -13.202127659574472, 7.797872340425528, -8.202127659574472, -16.202127659574472, -11.202127659574472, 0.7978723404255277, 1.7978723404255277, 15.797872340425528, -8.202127659574472, -9.202127659574472, 3.7978723404255277, -19.202127659574472, 3.7978723404255277, 5.797872340425528, -2.2021276595744723, 9.797872340425528, 7.797872340425528, -5.202127659574472, -8.202127659574472, 2.7978723404255277, -12.202127659574472, 9.797872340425528, -14.202127659574472, -13.202127659574472, 12.797872340425528, 1.7978723404255277, 13.797872340425528, -2.2021276595744723, -4.202127659574472, 3.7978723404255277, -7.202127659574472, 11.797872340425528, 2.7978723404255277, 17.797872340425528, 10.797872340425528, -11.202127659574472, -5.202127659574472, 8.797872340425528, 8.797872340425528, -4.202127659574472, -10.202127659574472, -0.20212765957447232, -9.202127659574472, -5.202127659574472, -2.2021276595744723, 12.797872340425528, 15.797872340425528, -6.202127659574472, -7.202127659574472, 1.7978723404255277, -5.202127659574472, 0.7978723404255277, 12.797872340425528, 4.797872340425528, -2.2021276595744723, 8.797872340425528, -11.202127659574472, -12.202127659574472, 22.797872340425528, 6.797872340425528, 17.797872340425528, -19.202127659574472, 7.797872340425528, 12.797872340425528, -11.202127659574472, 8.797872340425528, -14.202127659574472, 9.797872340425528, 4.797872340425528, -13.202127659574472, -3.2021276595744723, 11.797872340425528, -3.2021276595744723, 13.797872340425528, 8.797872340425528, -8.202127659574472, -3.2021276595744723, 8.797872340425528, -9.202127659574472, 2.7978723404255277, -7.202127659574472, 1.7978723404255277, -10.202127659574472, -7.202127659574472, 2.7978723404255277, -13.202127659574472, 7.797872340425528, -5.202127659574472, -5.202127659574472, -3.2021276595744723, -2.2021276595744723, 11.797872340425528, 5.797872340425528, -14.202127659574472, -12.202127659574472, -4.202127659574472, 8.797872340425528, 16.797872340425528, -0.20212765957447232, 18.797872340425528, -5.202127659574472, 5.797872340425528, 10.797872340425528, -2.2021276595744723, 6.797872340425528, -12.202127659574472, -4.202127659574472, 1.7978723404255277, -8.202127659574472, -8.202127659574472, -2.2021276595744723, 9.797872340425528, -14.202127659574472, -4.202127659574472, -16.202127659574472, 4.797872340425528, -19.202127659574472, -7.202127659574472, -0.20212765957447232, -7.202127659574472, -11.202127659574472, -10.202127659574472, 14.797872340425528, -16.202127659574472, 2.7978723404255277, -0.20212765957447232, 4.797872340425528, -15.202127659574472, 9.797872340425528, 5.797872340425528, 1.7978723404255277, -3.2021276595744723, -7.202127659574472, 14.797872340425528, -11.202127659574472, 3.7978723404255277, -5.202127659574472, 0.7978723404255277, 6.797872340425528, -7.202127659574472, 8.797872340425528, -4.202127659574472, -6.202127659574472, 1.7978723404255277, -17.202127659574472, -9.202127659574472, -5.202127659574472, -3.2021276595744723, -15.202127659574472, -19.202127659574472, 4.797872340425528, 8.797872340425528, -2.2021276595744723, -2.2021276595744723, 15.797872340425528, -8.202127659574472, 6.797872340425528, -14.202127659574472, 12.797872340425528, -6.202127659574472, -12.202127659574472, -1.2021276595744723, -22.202127659574472, -0.20212765957447232, -6.202127659574472, 5.797872340425528, 2.7978723404255277, -8.202127659574472, -4.202127659574472, 14.797872340425528, 3.7978723404255277, -7.202127659574472, -3.2021276595744723, -1.2021276595744723, -6.202127659574472, -2.2021276595744723, 4.797872340425528, 5.797872340425528, -7.202127659574472, 14.797872340425528, 0.7978723404255277, 2.7978723404255277, 10.797872340425528, -9.202127659574472, 10.797872340425528, 0.7978723404255277, -10.202127659574472, -0.20212765957447232, 1.7978723404255277, -4.202127659574472, 0.7978723404255277, -8.202127659574472, -17.202127659574472, 3.7978723404255277, -0.20212765957447232, -5.202127659574472, 0.7978723404255277, -13.202127659574472, 13.797872340425528, -6.202127659574472, 20.797872340425528, 1.7978723404255277, -3.2021276595744723, -1.2021276595744723, -4.202127659574472, -11.202127659574472, -10.202127659574472, -11.202127659574472, 0.7978723404255277, 2.7978723404255277, 7.797872340425528, -1.2021276595744723, 5.797872340425528, 9.797872340425528, -3.2021276595744723, 7.797872340425528, 5.797872340425528, -1.2021276595744723, -10.202127659574472, 3.7978723404255277, -12.202127659574472, 5.797872340425528, -3.2021276595744723, 0.7978723404255277, -0.20212765957447232, -2.2021276595744723, -9.202127659574472, 5.797872340425528, 2.7978723404255277, 1.7978723404255277, 9.797872340425528, -2.2021276595744723, -12.202127659574472, -0.20212765957447232, -7.202127659574472, 16.797872340425528, -12.202127659574472, -5.202127659574472, -0.20212765957447232, 4.797872340425528, 2.7978723404255277, -2.2021276595744723, 1.7978723404255277, -18.202127659574472, 17.797872340425528, 12.797872340425528, 5.797872340425528, -0.20212765957447232, -15.202127659574472, 4.797872340425528, 0.7978723404255277, -10.202127659574472, 1.7978723404255277, 0.7978723404255277, 7.797872340425528, -3.2021276595744723, -12.202127659574472, 0.7978723404255277, 1.7978723404255277, 9.797872340425528, -8.202127659574472, -1.2021276595744723, -22.202127659574472, -8.202127659574472, 3.7978723404255277, 14.797872340425528, -0.20212765957447232, -6.202127659574472, -1.2021276595744723, 8.797872340425528, 10.797872340425528, -2.2021276595744723, -0.20212765957447232, -0.20212765957447232, -13.202127659574472, -5.202127659574472, 1.7978723404255277, -2.2021276595744723, 20.797872340425528, -20.202127659574472, -2.2021276595744723, -10.202127659574472, -3.2021276595744723, 10.797872340425528, -7.202127659574472, 7.797872340425528, 7.797872340425528, 1.7978723404255277, -3.2021276595744723, -0.20212765957447232, -13.202127659574472, -3.2021276595744723, 16.797872340425528, 2.7978723404255277, 2.7978723404255277, -7.202127659574472, -2.2021276595744723, 5.797872340425528, -13.202127659574472, 10.797872340425528, -4.202127659574472, 7.797872340425528, -3.2021276595744723, -20.202127659574472, 15.797872340425528, -0.20212765957447232, 11.797872340425528, 9.797872340425528, -10.202127659574472, -1.2021276595744723, 1.7978723404255277, -7.202127659574472, -0.20212765957447232, 5.797872340425528, -15.202127659574472, 7.797872340425528, 5.797872340425528, -8.202127659574472, -7.202127659574472, 14.797872340425528, 2.7978723404255277, 2.7978723404255277, -3.2021276595744723, 0.7978723404255277, -18.202127659574472, 20.797872340425528, 9.797872340425528, 5.797872340425528, -20.202127659574472, 17.797872340425528, 11.797872340425528, -1.2021276595744723, 0.7978723404255277, -10.202127659574472, -8.202127659574472, 20.797872340425528, -7.202127659574472, -4.202127659574472, 11.797872340425528, -10.202127659574472, 2.7978723404255277, 5.797872340425528, 1.7978723404255277, -11.202127659574472, 8.797872340425528, -3.2021276595744723, -4.202127659574472, -1.2021276595744723, 6.797872340425528, 0.7978723404255277, -6.202127659574472, -2.2021276595744723, 1.7978723404255277, -7.202127659574472, -5.202127659574472, -2.2021276595744723, -4.202127659574472, -3.2021276595744723, -7.202127659574472, 7.797872340425528, 7.797872340425528, -16.202127659574472, -6.202127659574472, 6.797872340425528, -0.20212765957447232, 2.7978723404255277, 17.797872340425528, 10.797872340425528, -17.202127659574472, -9.202127659574472, 6.797872340425528, 14.797872340425528, 4.797872340425528, -7.202127659574472, 13.797872340425528, 18.797872340425528, 12.797872340425528, 2.7978723404255277, 9.797872340425528, 4.797872340425528, 10.797872340425528, -12.202127659574472, -4.202127659574472, -15.202127659574472, -3.2021276595744723, -3.2021276595744723, -5.202127659574472, -3.2021276595744723, -9.202127659574472, -3.2021276595744723, -18.202127659574472, 5.797872340425528, -3.2021276595744723, -2.2021276595744723, -12.202127659574472, -19.202127659574472, -0.20212765957447232, 5.797872340425528, 0.7978723404255277, -0.20212765957447232, -4.202127659574472, -0.20212765957447232, 17.797872340425528, 6.797872340425528, -8.202127659574472, -7.202127659574472, -6.202127659574472, -16.202127659574472, 11.797872340425528, -7.202127659574472, -1.2021276595744723, 1.7978723404255277, 3.7978723404255277, -19.202127659574472, -0.20212765957447232, -1.2021276595744723, -12.202127659574472, -5.202127659574472, 0.7978723404255277, -1.2021276595744723, 4.797872340425528, 2.7978723404255277, -12.202127659574472, 13.797872340425528, 15.797872340425528, 3.7978723404255277, 3.7978723404255277, 19.797872340425528, 7.797872340425528, -3.2021276595744723, -5.202127659574472, 1.7978723404255277, 0.7978723404255277, -4.202127659574472, 9.797872340425528, -12.202127659574472, 8.797872340425528, -1.2021276595744723, 9.797872340425528, 4.797872340425528, 1.7978723404255277, -12.202127659574472, -2.2021276595744723, 14.797872340425528, -0.20212765957447232, -4.202127659574472, -14.202127659574472, -0.20212765957447232, 11.797872340425528, 14.797872340425528, -2.2021276595744723, 8.797872340425528, -3.2021276595744723, -8.202127659574472, -16.202127659574472, 3.7978723404255277, -10.202127659574472, 8.797872340425528, 4.797872340425528, -0.20212765957447232, 5.797872340425528, 5.797872340425528, 0.7978723404255277, -12.202127659574472, -8.202127659574472, 0.7978723404255277, 13.797872340425528, -1.2021276595744723, -15.202127659574472, -7.202127659574472, 3.7978723404255277, 8.797872340425528, -0.20212765957447232, -3.2021276595744723, 7.797872340425528, 12.797872340425528, 7.797872340425528, 12.797872340425528, 6.797872340425528, -2.2021276595744723, -0.20212765957447232, -16.202127659574472, 3.7978723404255277, 4.797872340425528, 19.797872340425528, -0.20212765957447232, -5.202127659574472, -2.2021276595744723, 0.7978723404255277, -8.202127659574472, -2.2021276595744723, 9.797872340425528, -6.202127659574472, -7.202127659574472, -15.202127659574472, -3.2021276595744723, 14.797872340425528, 5.797872340425528, -6.202127659574472, 7.797872340425528, 2.7978723404255277, 4.797872340425528, -6.202127659574472, -7.202127659574472, 8.797872340425528, 10.797872340425528, -8.202127659574472, -8.202127659574472, 2.7978723404255277, 2.7978723404255277, 5.797872340425528, -5.202127659574472, -13.202127659574472, -21.202127659574472, -3.2021276595744723, 1.7978723404255277, -7.202127659574472, -0.20212765957447232, -9.202127659574472, -3.2021276595744723, -4.202127659574472, -6.202127659574472, -5.202127659574472, 14.797872340425528, -1.2021276595744723, 20.797872340425528, 1.7978723404255277, -17.202127659574472]] caption="Corrected Signal"
  out "Max. Rep. Rate (Hz)":dbl=7091.695624423801
  out "Data Collection Time per Column":dbl=2.00004285
  out "Minimum Sync Pulse Period(µs)":dbl=141.01 format="%.2f"
  in  "y units":u16(ring) items=["Bin #", "Sampling Time(µs)", "Range(m)"]
  in  "Time Resolution Per Bin(ns)":u16=250 min=5 max=1063 step=1
  in  "Number of Accumulates":u32=14285 min=1 max=32767 step=1
  in  "Pulse A Polarity":enum16{"Low", "High"}(ring)=enum."High"
  in  "Sync Pulse Polarity":enum32{"Low", "High"}(ring)=enum."High"
  in  "Accumulation Delay(ns)":u16=10 min=10 max=1270 step=1
  in  "Pulse B Delay(ns)":u32=80 min=80 max=327600 step=1
  in  "Pulse A Delay(ns)":u32=80 min=80 max=327600
  in  "bins":u32=560 min=2 max=4095 step=1
  out "y offset":u16=10
  in  "ns scale":u16=250
  in  "Pulse B Polarity":enum16{"Low", "High"}(ring)=enum."High"
  out "Running?":bool
  out "Device ID":u32
  out "Open?":bool=TRUE
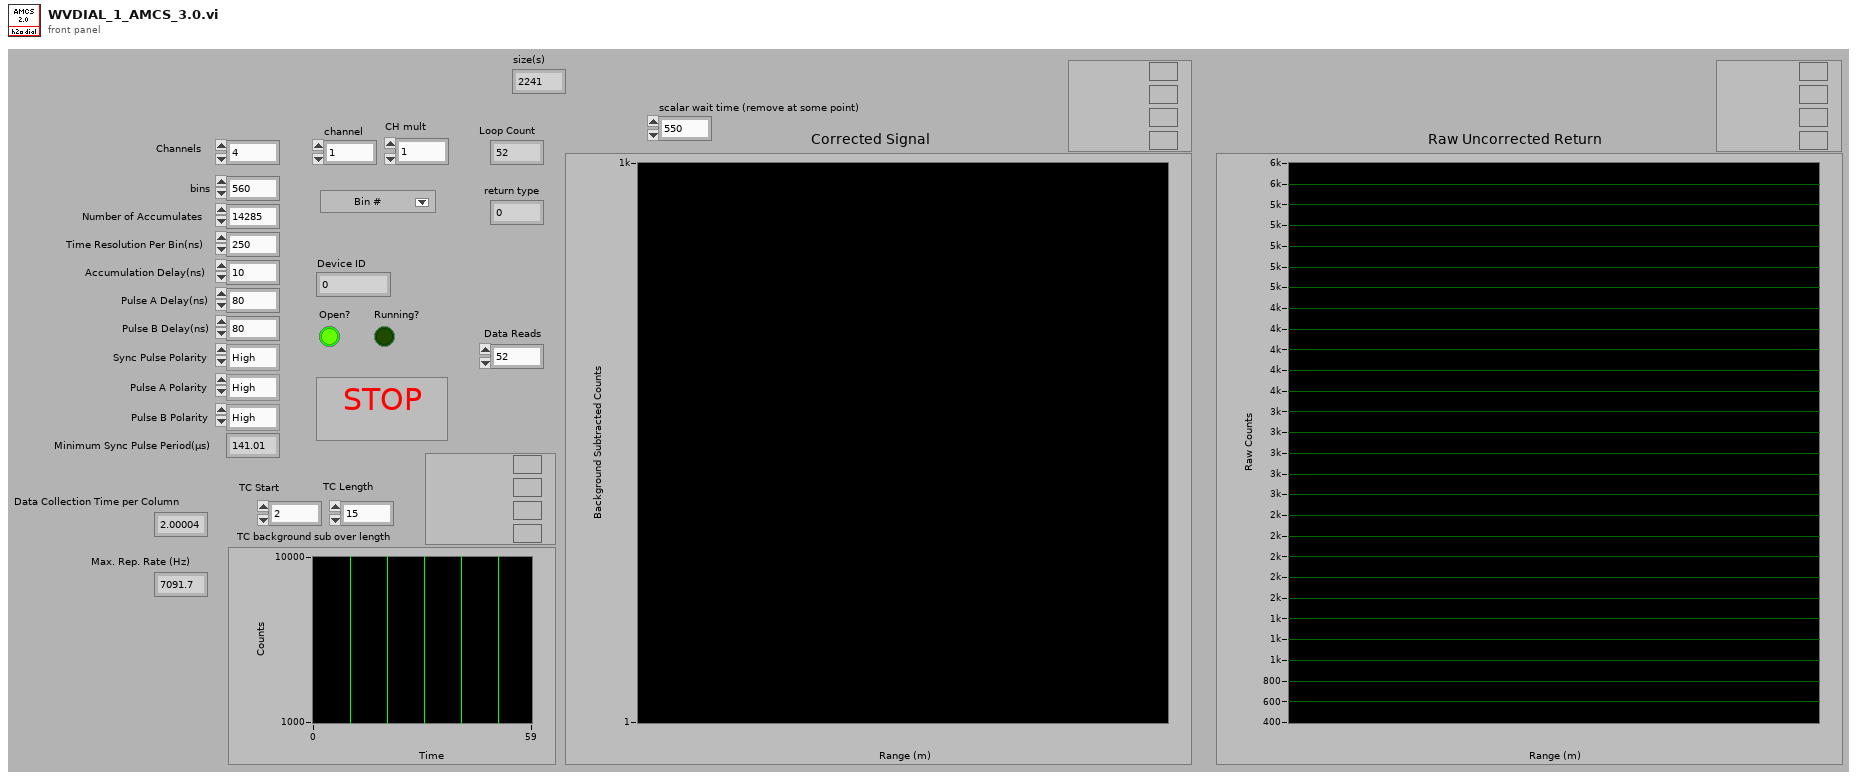
[diagram p1: front panel]
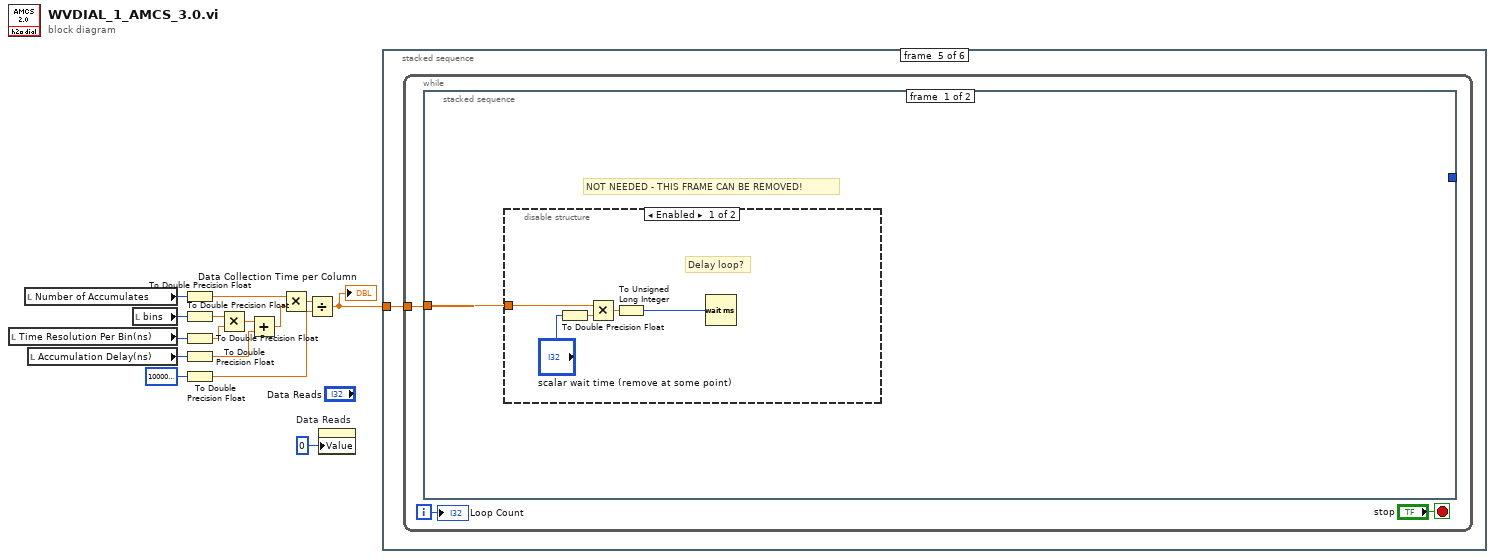
[diagram p0: block diagram]
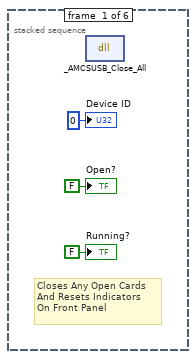
[diagram p2: hidden frame]
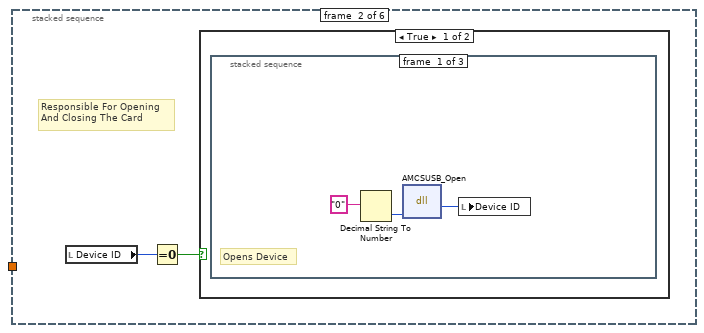
[diagram p3: hidden frame]
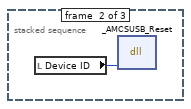
[diagram p4: hidden frame]
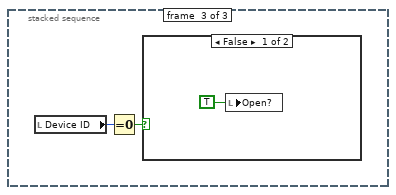
[diagram p5: hidden frame]
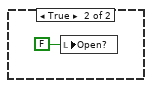
[diagram p6: hidden frame]
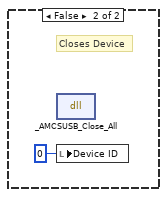
[diagram p7: hidden frame]
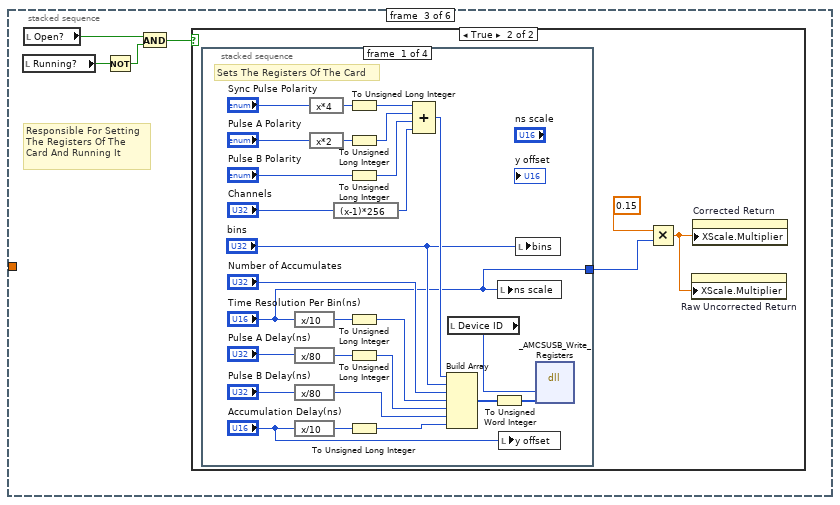
[diagram p8: hidden frame]
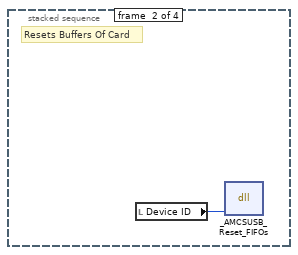
[diagram p10: hidden frame]
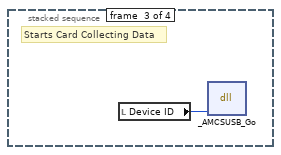
[diagram p11: hidden frame]
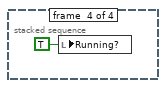
[diagram p12: hidden frame]
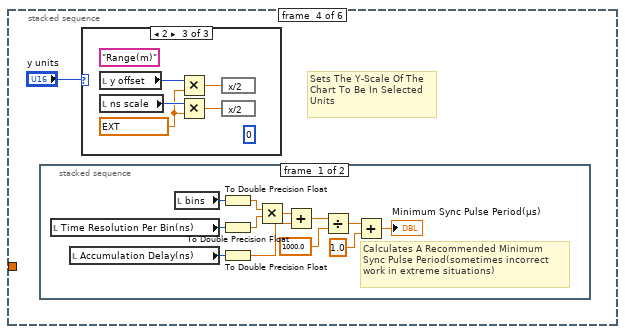
[diagram p13: hidden frame]
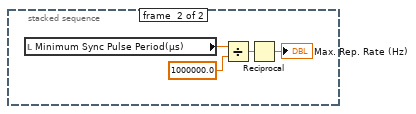
[diagram p14: hidden frame]
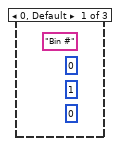
[diagram p15: hidden frame]
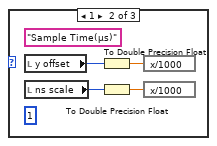
[diagram p16: hidden frame]
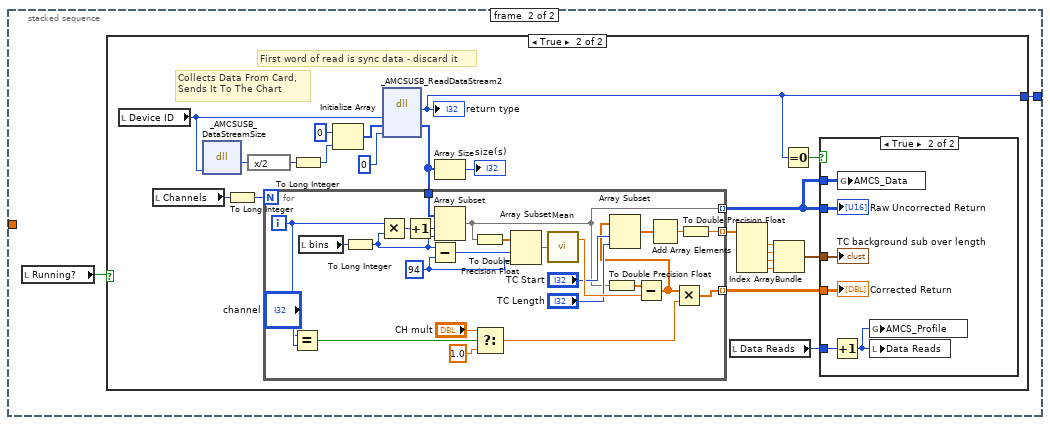
[diagram p18: hidden frame]
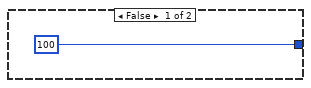
[diagram p19: hidden frame]
diagram:
  n1 = local read "Time Resolution Per Bin(ns)"() -> (w4:u16)
  n2 = local read "Number of Accumulates"() -> (w11:u32)
  n3 = local read "Accumulation Delay(ns)"() -> (w2:u16)
  n4 = local read "bins"() -> (w6:u32)
  n5 = To Double Precision Float(number=w11) -> (double precision float=w10:dbl)
  n6 = To Double Precision Float(number=w6) -> (double precision float=w5:dbl)
  n7 = To Double Precision Float(number=w4) -> (double precision float=w7:dbl)
  n8 = To Double Precision Float(number=w2) -> (double precision float=w3:dbl)
  n9 = To Double Precision Float(number=1000000000) -> (double precision float=w8:dbl)
  n10 = Multiply(x=w5, y=w7) -> (x*y=w15:dbl)
  n11 = Add(x=w15, y=w3) -> (x+y=w14:dbl)
  n12 = Multiply(x=w10, y=w14) -> (x*y=w13:dbl)
  n13 = Divide(x=w13, y=w8) -> (x/y=w12:dbl)
  "Data Collection Time per Column" <- w12
  n14 = property on="Data Reads" class="DigNum (strict)"("Value"=0 ("Data Reads")) -> ()  [unwired: 2 in, 2 out]
  n15 = stacked-sequence {
    tunnel: w12 -> [_ _ _ _ w93 _]
    frame #0 {
      # "Closes Any Open Cards\nAnd Resets Indicators\nOn Front Panel"
      n16 = dll-call lib="AmcsUsb.dll" fn="_AMCSUSB_Close_All" label="Close_All"() -> ()  [unwired: 4 in, 2 out]
      "Open?" <- FALSE ("Open?")
      "Device ID" <- u32 0 ("Device ID")
      "Running?" <- FALSE ("Running?")
    }
    frame #1 {
      # "Responsible For Opening\nAnd Closing The Card"
      n17 = local read "Device ID"() -> (w20:u32)
      n18 = Equal To 0?(x=w20) -> (x = 0?=w19:bool)
      n19 = case shown="True" w19 {
        frame True {
          # "Opens Device"
          n20 = stacked-sequence {
            frame #0 {
              n21 = Decimal String To Number(string="0" ("Device Number")) -> (number=w21:i32)  [unwired: 2 in, 1 out]
              n22 = dll-call lib="AmcsUsb.dll" fn="AMCSUSB_Open"("devnum"=w21) -> ("return type"=w22:u32)  [unwired: 4 in, 2 out]
              n23 = local write "Device ID"(w22) -> ()
            }
            frame #1 {
              n24 = local read "Device ID"() -> (w24:u32)
              n25 = dll-call lib="AmcsUsb.dll" fn="_AMCSUSB_Reset" label="Reset"("handle"=w24) -> ()  [unwired: 5 in, 2 out]
            }
            frame #2 {
              n26 = local read "Device ID"() -> (w25:u32)
              n27 = Equal To 0?(x=w25) -> (x = 0?=w26:bool)
              n28 = case shown="False" w26 {
                frame False {
                  n29 = local write "Open?"(TRUE ("Open?")) -> ()
                }
                frame True {
                  n30 = local write "Open?"(FALSE ("Open?")) -> ()
                }
              }
            }
          }
        }
        frame False {
          # "Closes Device"
          n31 = dll-call lib="AmcsUsb.dll" fn="_AMCSUSB_Close_All" label="Close_All"() -> ()  [unwired: 4 in, 2 out]
          n32 = local write "Device ID"(u32 0 ("Device ID")) -> ()
        }
      }
    }
    frame #2 {
      # "Responsible For Setting\nThe Registers Of The\nCard And Running It"
      n33 = local read "Running?"() -> (w32:bool)
      n34 = local read "Open?"() -> (w33:bool)
      n35 = Not(x=w32) -> (.not. x?=w31:bool)
      n36 = And(x=w33, y=w31) -> (x .and. y?=w30:bool)
      n37 = case shown="True" w30 {
        frame False {
        }
        frame True {
          n38 = stacked-sequence {
            tunnel: ["Time Resolution Per Bin(ns)" _ _ _] -> w35
            frame #0 {
              # "Sets The Registers Of The Card"
              n39 = expression code="x/10"("Time Resolution Per Bin(ns)") -> (w43:u16)
              n40 = expression code="x/80"("Pulse A Delay(ns)") -> (w45:u32)
              n41 = expression code="x/80"("Pulse B Delay(ns)") -> (w63:u32)
              n42 = expression code="x/10"("Accumulation Delay(ns)") -> (w47:u16)
              n43 = expression code="x*4"("Sync Pulse Polarity") -> (w52:enum32{"Low", "High"})
              n44 = expression code="x*2"("Pulse A Polarity") -> (w51:enum16{"Low", "High"})
              n45 = expression code="(x-1)*256"("Channels") -> (w57:u32)
              n46 = To Unsigned Long Integer(number=w52) -> (unsigned 32bit integer=w53:u32)
              n47 = To Unsigned Long Integer(number=w51) -> (unsigned 32bit integer=w50:u32)
              n48 = To Unsigned Long Integer(number="Pulse B Polarity") -> (unsigned 32bit integer=w48:u32)
              n49 = To Unsigned Long Integer(number=w43) -> (unsigned 32bit integer=w42:u32)
              n50 = To Unsigned Long Integer(number=w45) -> (unsigned 32bit integer=w44:u32)
              n51 = To Unsigned Long Integer(number=w47) -> (unsigned 32bit integer=w46:u32)
              n52 = Compound Arithmetic op=ADD(w53, w50, w48, w57) -> (w62:u32)
              n53 = Build Array(w62, "bins", "Number of Accumulates", w42, w44, w63, w46) -> (w41:u32[])
              n54 = local read "Device ID"() -> (w56:u32)
              n55 = To Unsigned Word Integer(number=w41) -> (unsigned 16bit integer=w40:u16[])
              n56 = local write "ns scale"("Time Resolution Per Bin(ns)") -> ()
              n57 = local write "y offset"("Accumulation Delay(ns)") -> ()
              n58 = local write "bins"("bins") -> ()
              n59 = dll-call lib="AmcsUsb.dll" fn="_AMCSUSB_Write_Registers" label="Write_Registers"("handle"=w56, "registers"=w40) -> ()  [unwired: 6 in, 2 out]
            }
            frame #1 {
              # "Resets Buffers Of Card"
              n60 = local read "Device ID"() -> (w64:u32)
              n61 = dll-call lib="AmcsUsb.dll" fn="_AMCSUSB_Reset_FIFOs" label="Reset_FIFOs"("handle"=w64) -> ()  [unwired: 5 in, 2 out]
            }
            frame #2 {
              # "Starts Card Collecting Data"
              n62 = local read "Device ID"() -> (w65:u32)
              n63 = dll-call lib="AmcsUsb.dll" fn="_AMCSUSB_Go" label="Go"("handle"=w65) -> ()  [unwired: 5 in, 2 out]
            }
            frame #3 {
              n64 = local write "Running?"(TRUE) -> ()
            }
          }
          n65 = Multiply(x=0.15, y=w35) -> (x*y=w34:dbl)
          n66 = property on="Raw Uncorrected Return" class="WFGraph (strict)"("XScale.Multiplier"=w34) -> ()  [unwired: 2 in, 2 out]
          n67 = property on="Corrected Return" class="WFGraph (strict)"("XScale.Multiplier"=w34) -> ()  [unwired: 2 in, 2 out]
        }
      }
    }
    frame #3 {
      # "Sets The Y-Scale Of The\nChart To Be In Selected\nUnits"
      n68 = stacked-sequence {
        frame #0 {
          # "Calculates A Recommended Minimum\nSync Pulse Period(sometimes incorrect\nwork in extreme situations)"
          n69 = local read "Time Resolution Per Bin(ns)"() -> (w74:u16)
          n70 = local read "Accumulation Delay(ns)"() -> (w76:u16)
          n71 = local read "bins"() -> (w75:u32)
          n72 = To Double Precision Float(number=w75) -> (double precision float=w77:dbl)
          n73 = To Double Precision Float(number=w74) -> (double precision float=w78:dbl)
          n74 = To Double Precision Float(number=w76) -> (double precision float=w79:dbl)
          n75 = Multiply(x=w77, y=w78) -> (x*y=w73:dbl)
          n76 = Add(x=w73, y=w79) -> (x+y=w71:dbl)
          n77 = Divide(x=w71, y=1000.0) -> (x/y=w70:dbl)
          n78 = Add(x=w70, y=1.0) -> (x+y=→"Minimum Sync Pulse Period(µs)":dbl)
        }
        frame #1 {
          n79 = local read "Minimum Sync Pulse Period(µs)"() -> (w81:dbl)
          n80 = Divide(x=w81, y=1000000.0) -> (x/y=w80:dbl)
          n81 = Reciprocal(x=w80) -> (1/x=→"Max. Rep. Rate (Hz)":dbl)
        }
      }
      n82 = case shown="2" "y units" {
        frame 0, Default {
          (unwired) u8 0 ("Y Scale.Format & Precision:Precision")
          (unwired) u16 1 ("Y Scale.Offset and Multiplier:Multiplier")
          (unwired) "Bin #" ("Y Scale.Name Label.Text")
          (unwired) u16 0 ("Y Scale.Offset and Multiplier:Offset")
        }
        frame 1 {
          (unwired) u8 1 ("Y Scale.Format & Precision:Precision")
          (unwired) "Sample Time(µs)" ("Y Scale.Name Label.Text")
          n83 = local read "y offset"() -> (w87:u16)
          n84 = local read "ns scale"() -> (w86:u16)
          n85 = To Double Precision Float(number=w87) -> (double precision float=w85:dbl)
          n86 = To Double Precision Float(number=w86) -> (double precision float=w84:dbl)
          n87 = expression code="x/1000"(w85) -> ()  [unwired: 1 out]
          n88 = expression code="x/1000"(w84) -> ()  [unwired: 1 out]
        }
        frame 2 {
          (unwired) u8 0 ("Y Scale.Format & Precision:Precision")
          w88 = ext 0.299792458 ("y")
          (unwired) "Range(m)" ("Y Scale.Name Label.Text")
          n89 = local read "y offset"() -> (w91:u16)
          n90 = local read "ns scale"() -> (w92:u16)
          n91 = Multiply(x=w91, y=w88) -> (x*y=w90:ext)
          n92 = Multiply(x=w92, y=w88) -> (x*y=w89:ext)
          n93 = expression code="x/2"(w90) -> ()  [unwired: 1 out]
          n94 = expression code="x/2"(w89) -> ()  [unwired: 1 out]
        }
      }
    }
    frame #4 {
      n95 = while {
        tunnel: w93 -> [w96]
        i -> [w94]
        stop <- "stop" stop-if-true
        n96 = stacked-sequence {
          tunnel: w96 -> [w97 _]
          tunnel: [_ w104] -> _
          frame #0 {
            # "NOT NEEDED - THIS FRAME CAN BE REMOVED!"
            n97 = disable-structure shown="Enabled" {
              disable-tunnel: w97 -> [w102 _]
              frame Enabled {
                # "Delay loop?"
                n98 = To Double Precision Float(number="scalar wait time (remove at some point)") -> (double precision float=w100:dbl)
                n99 = Multiply(x=w102, y=w100) -> (x*y=w99:dbl)
                n100 = To Unsigned Long Integer(number=w99) -> (unsigned 32bit integer=w98:u32)
                n101 = Wait (ms)(milliseconds to wait=w98) -> ()  [unwired: 1 out]
              }
              frame Disabled {
              }
            }
          }
          frame #1 {
            n102 = local read "Running?"() -> (w103:bool)
            n103 = case shown="True" w103 {
              tunnel: [100 ("return type") w112] -> w104
              frame False {
              }
              frame True {
                # "First word of read is sync data - discard it"
                # "Collects Data From Card,\nSends It To The Chart"
                n104 = local read "Device ID"() -> (w124:u32)
                n105 = local read "Channels"() -> (w116:u32)
                n106 = dll-call lib="AmcsUsb.dll" fn="_AMCSUSB_DataStreamSize" label="DataStreamSize"("handle"=w124) -> ("return type"=w123:u16)  [unwired: 4 in, 2 out]
                n107 = To Long Integer(number=w116) -> (32bit integer=w117:i32)
                n108 = expression code="x/2"(w123) -> (w122:u16)
                n109 = To Long Integer(number=w122) -> (32bit integer=w121:i32)
                n110 = Initialize Array(u32 0 ("element"), w121) -> (w125:u32[])
                n111 = dll-call lib="AmcsUsb.dll" fn="_AMCSUSB_ReadDataStream2" label="ReadDataStream2"("handle"=w124, "buffer"=w125, "BytesReturned"=u32 0) -> ("return type"=w112:i32, "buffer"=w111:u16[])  [unwired: 5 in, 2 out]
                "return type" <- w112
                n112 = for {
                  N: w117 -> [_]
                  tunnel: [w136] -> w115 mode=indexing
                  tunnel: [w135] -> w120 mode=indexing
                  tunnel: [w138] -> w109 mode=indexing
                  tunnel: w111 -> [w142]
                  i -> [w129]
                  w144 = 94 ("y")
                  n113 = Equal?(x=w129, y="channel") -> (x = y?=w133:bool)
                  n114 = local read "bins"() -> (w148:u32)
                  n115 = To Long Integer(number=w148) -> (32bit integer=w146:i32)
                  n116 = Multiply(x=w129, y=w146) -> (x*y=w147:i32)
                  n117 = Increment(x=w147) -> (x+1=w141:i32)
                  n118 = Subtract(x=w146, y=w144) -> (x-y=w145:i32)
                  n119 = Array Subset(array=w142, index=w141, length=w146) -> (w138:u16[])
                  n120 = To Double Precision Float(number=w138) -> (double precision float=w137:dbl[])
                  n121 = Select(t="CH mult", s=w133, f=1.0 ("y")) -> (s? t:f=w130:dbl)
                  n122 = Array Subset(array=w137, index=w145, length=w144) -> (w152:dbl[])
                  n123 = call-poly <vilib>:"Mean.vi"("X"=w152) -> ("mean"=w150:dbl)  [unwired: 1 out]
                  n124 = To Double Precision Float(number=w138) -> (double precision float=w149:dbl[])
                  n125 = Subtract(x=w149, y=w150) -> (x-y=w128:dbl[])
                  n126 = Array Subset(array=w128, index="TC Start", length="TC Length") -> (w151:dbl[])
                  n127 = Add Array Elements(numeric array=w151) -> (sum=w143:dbl)
                  n128 = Multiply(x=w128, y=w130) -> (x*y=w135:dbl[])
                  n129 = To Double Precision Float(number=w143) -> (double precision float=w136:dbl)
                }
                n130 = Array Size(array=w111) -> (size(s)=→"size(s)":i32)
                n131 = local read "Data Reads"() -> (w108:i32)
                n132 = Index Array(array=w115) -> (element #1=w107:dbl, element #2=w106:dbl, element #3=w114:dbl, element #4=w113:dbl)  [unwired: 4 in]
                n133 = Bundle(w107, w106, w114, w113) -> (w118:cluster{dbl, dbl, dbl, dbl})  [unwired: 1 in]
                n134 = Equal To 0?(x=w112) -> (x = 0?=w119:bool)
                n135 = case shown="True" w119 {
                  tunnel: w120 -> [_ w158]
                  tunnel: w109 -> [_ w157]
                  tunnel: w118 -> [_ w156]
                  tunnel: w109 -> [_ w155]
                  tunnel: w108 -> [_ w154]
                  frame False {
                  }
                  frame True {
                    n136 = Increment(x=w154) -> (x+1=w153:i32)
                    n137 = global write "AMCS_Data.vi" "AMCS_Data"(w155) -> ()
                    n138 = global write "AMCS_Data.vi" "AMCS_Profile"(w153) -> ()
                    n139 = local write "Data Reads"(w153) -> ()
                    "Corrected Return" <- w158
                    "Raw Uncorrected Return" <- w157
                    "TC background sub over length" <- w156
                  }
                }
              }
            }
          }
        }
        "Loop Count" <- w94
      }
    }
    frame #5 {
      # "Closes Any Open Cards\nAnd Resets Indicators\nOn Front Panel"
      n140 = dll-call lib="AmcsUsb.dll" fn="_AMCSUSB_Close_All" label="Close_All"() -> ()  [unwired: 4 in, 2 out]
      n141 = local write "Device ID"(u32 0 ("Device ID")) -> ()
      n142 = local write "Open?"(TRUE ("Open?")) -> ()
      n143 = local write "Running?"(FALSE ("Running?")) -> ()
    }
  }
